vi "Memory.Pointer.Compare Size.vi"(8 "error in (no error)":errorcluster, 10 "Pointer b in":refnum<class "Memory.Pointer.lvclass">, 11 "Pointer a in":refnum<class "Memory.Pointer.lvclass">) -> (0 "error out":errorcluster, 1 "equal size?":bool, 2 "Pointer b out":refnum<class "Memory.Pointer.lvclass">, 3 "Pointer a out":refnum<class "Memory.Pointer.lvclass">)   [LabVIEW 2016, in "Memory.lvlib" / "Memory.Pointer.lvclass"]
uses:
  Memory.Pointer.lvclass
  Memory.Pointer.lvclass/Memory.Pointer.ctl
  Memory.Pointer.Errors.Size Mismatch.vi
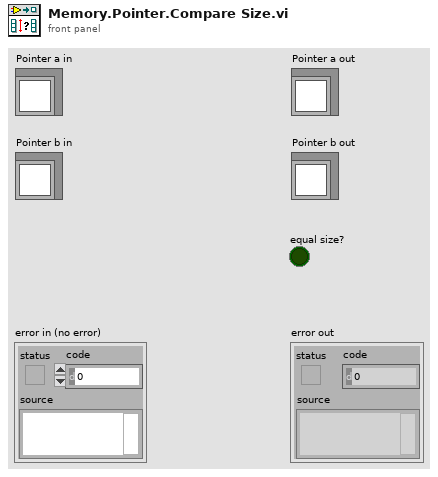
[diagram p1: front panel]
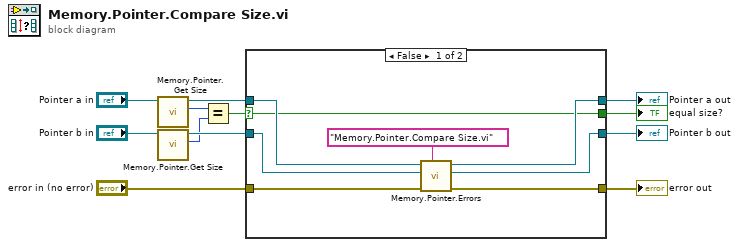
[diagram p0: block diagram]
diagram:
  n1 = call "Memory.Pointer.Get Size.vi"("Pointer in"="Pointer a in") -> ("size"=w10:u64, "Pointer out"=w9:refnum<class "Memory.Pointer.lvclass">)  [unwired: 9 in]
  n2 = call "Memory.Pointer.Get Size.vi"("Pointer in"="Pointer b in") -> ("size"=w6:u64, "Pointer out"=w8:refnum<class "Memory.Pointer.lvclass">)  [unwired: 9 in]
  n3 = Equal?(x=w10, y=w6) -> (x = y?=w7:bool)
  n4 = case shown="False" w7 {
    selector: w7 -> [w14 w22]
    tunnel: w9 -> [w17 w24]
    tunnel: w8 -> [w13 w23]
    tunnel: "error in (no error)" -> [w19 w21]
    tunnel: [w18 w21] -> w4
    tunnel: [w15 w24] -> w3
    tunnel: [w16 w23] -> w2
    tunnel: [w14 w22] -> w1
    frame False {
      n5 = call-poly "Memory.Pointer.Errors.vi"("error source vi name"="Memory.Pointer.Compare Size.vi" ("source vi name"), "error in (no error)"=w19, "Pointer b in"=w13, "Pointer a in"=w17) -> ("error out"=w18:errorcluster, "Pointer b out"=w16:refnum<class "Memory.Pointer.lvclass">, "Pointer a out"=w15:refnum<class "Memory.Pointer.lvclass">)  [unwired: 5 in]
    }
    frame True {
    }
  }
  "error out" <- w4
  "equal size?" <- w1
  "Pointer a out" <- w3
  "Pointer b out" <- w2
